vi "RoomPost.vi"(7 "LabVIEW Web Service Request":refnum<class "Web Request.lvclass">) -> ()   [LabVIEW 2015]
uses:
  <vilib>/wsapi/Web Request.lvclass
  TypeDef/RoomsActionEnum.ctl
panel:
  in  "Command":string
  out "request variables":cluster{"Key":string[], "Value":string[]}
  out "postdata":string
  out "Response":string
  in  "Room":i32
  # "Use the Web Service Request input terminal to call the VIs on the Web Services palette. Do not remove it from the connector pane unless you don't need access to the palette."
  # "Each additional control wired to the connector pane will be available as an input in the URL. To include an indicator in terminal-mode output (the default setting), it must also be wired to the connector pane."
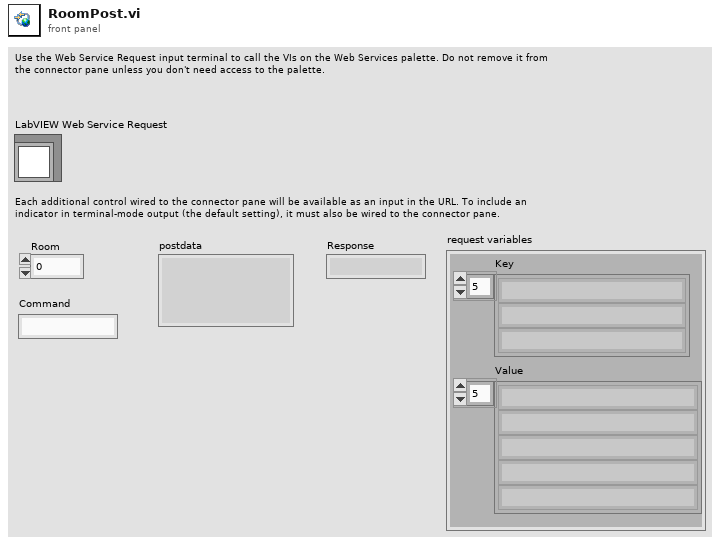
[diagram p1: front panel]
types:
  T1 = typedef "RoomsActionEnum.ctl" = enum16{"Init", "Add Room", "Remove Room", "Read Room", "Read Flag", "Read Flag State", "Write Flag State", "Read Flag Color", "Write Flag Color", "Read Bed Vacant", "Write Bed Vacant", "Read Personnel", "Add Personnel", "Remove Personnel", "Read Requests", "Add Request", "Remove Request", "Read Beacon ID", "Write Beacon ID", "Write Bed URL", "Read Bed URL"}
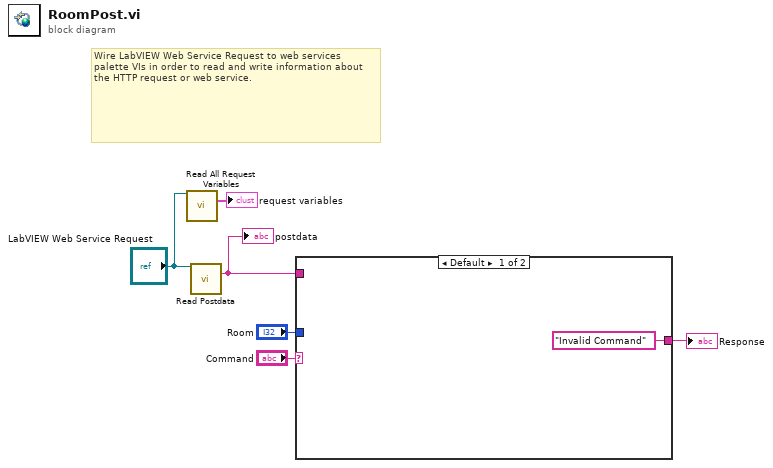
[diagram p0: block diagram]
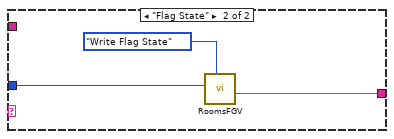
[diagram p2: hidden frame]
diagram:
  # "Wire LabVIEW Web Service Request to web services palette VIs in order to read and write information about the HTTP request or web service."
  n1 = call <vilib>:"Read All Request Variables.vi"("LabVIEW Web Service Request"="LabVIEW Web Service Request") -> ("request variables"=→"request variables":cluster{"Key":string[], "Value":string[]})  [unwired: 12 in, 2 out]
  n2 = call <vilib>:"Read Postdata.vi"("LabVIEW Web Service Request"="LabVIEW Web Service Request") -> ("postdata"=w3:string)  [unwired: 12 in, 2 out]
  "postdata" <- w3
  n3 = case shown="Default" "Command" {
    tunnel: w3 -> [_ _]
    tunnel: ["Invalid Command" ("Data Out") w9] -> w2
    tunnel: "Room" -> [_ w8]
    frame Default {
    }
    frame "Flag State" {
      n4 = call "RoomsFGV.vi"("Actions"=RoomsActionEnum."Write Flag State", "Room"=w8) -> ("Data Out"=w9:string)  [unwired: 8 in, 1 out]
    }
  }
  "Response" <- w2
